vi "SelectAndResizeImageForFitting.vi"(0 "IMAQ Actual Image":T3, 1 "IMAQ Fitting Image":T3, 2 "ImageDisplay Refnum":refnum<vi>, 3 "Select Gaussian \nFit Methode":T1(ring), 4 "Subsampling":i32(ring)=16 items=["1"=1, "2"=2, "4"=4, "8"=8, "16"=16], 5 "error in":errorcluster, 6 "SimulationParameters":dbl[](array[slide])=[97.19626168224299, 38.62928348909657, 51.09034267912772, 14.330218068535824, 24.922118380062305, 127.10280373831775] caption="Amplitude\n\n\nX-Position\n\n\nY-Position\n\n\nWidth A\n\n\nWidth B\n\n\nAngle" scale=0.0..200.0, 7 "Cyclic Calculation Refnum":refnum<vi>, 9 "Image Busy Refnum":refnum<vi>) -> (13 "disable fit":bool, 14 "IMAQ Fitting Image Out":T3, 15 "FittingImageArray":dbl[][](array[numeric]), 16 "X samples":i32, 17 "Y samples":i32, 18 "ROI Offset":i32[](array[numeric]), 19 "error out":errorcluster)   [LabVIEW 2015]
uses:
  <vilib>/vision/Image Controls.llb/IMAQ Image.ctl
  <vilib>/vision/NI_Vision_Development_Module.lvlib
panel:
  out "ROI":T2
  in  "num X samples":i32=120
  in  "num Y samples":i32=100
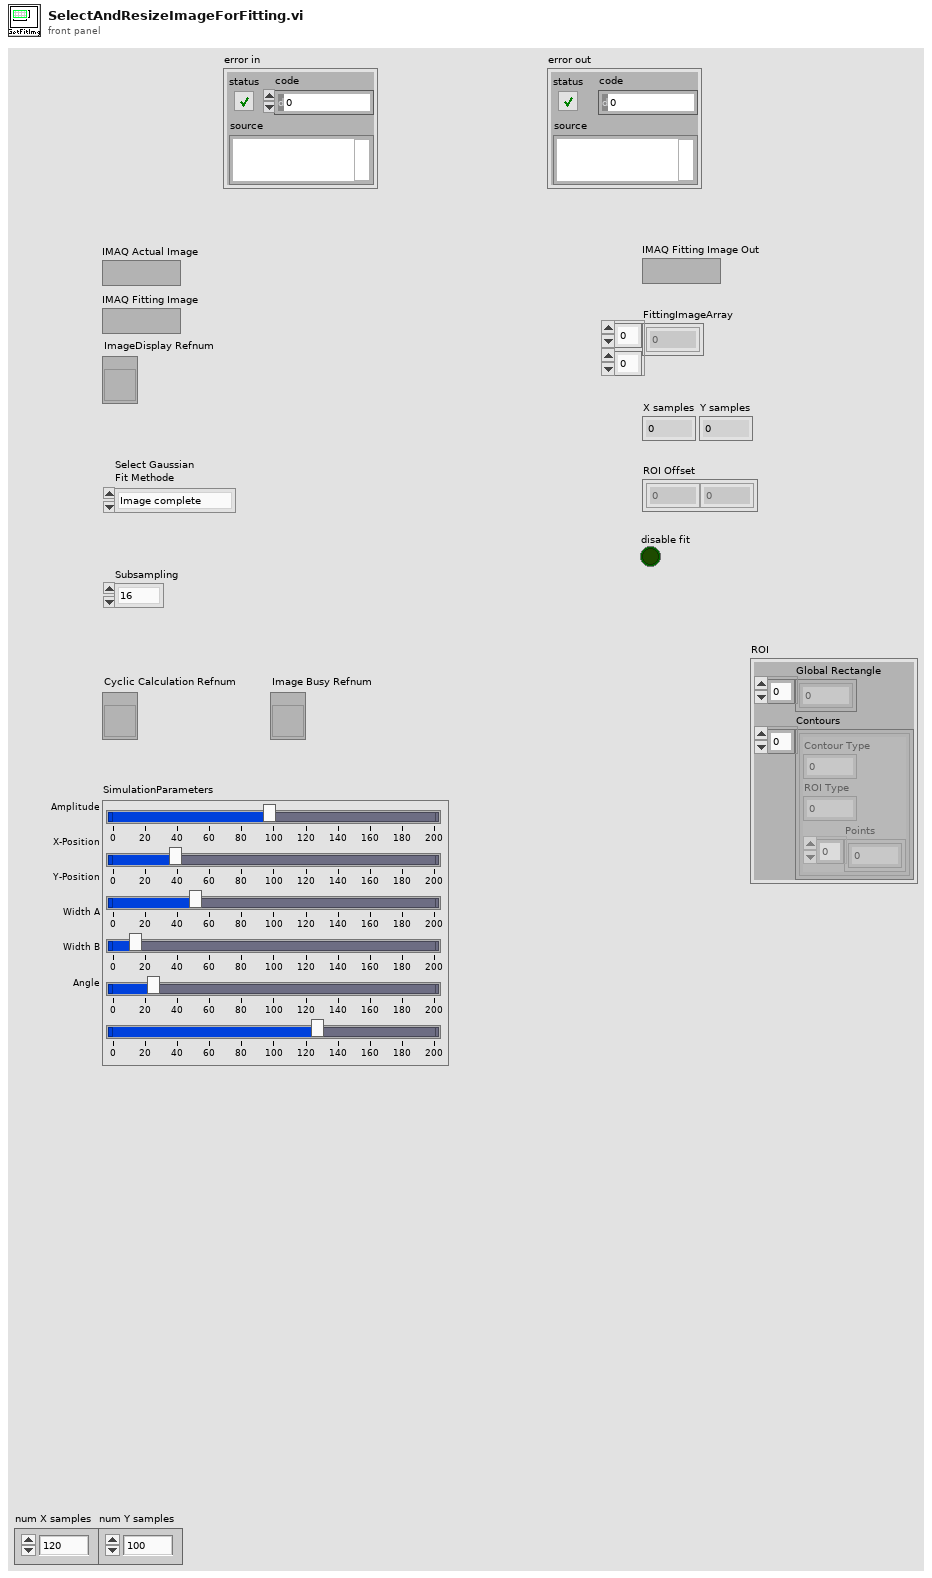
[diagram p1: front panel]
types:
  T1 = enum16{"Image complete", "Image with ROI", "AutoROI", "Simulation"}
  T2 = cluster{"Global Rectangle":i32[], "Contours":cluster{"Contour Type":u32, "ROI Type":u32, "Points":i32[]}[]}
  T3 = typedef "IMAQ Image.ctl" = refnum<image>
  T4 = typedef "IMAQ Rectangle" = cluster{"Left":i32, "Top":i32, "Right":i32, "Bottom":i32, "Rotation":dbl}
  T5 = cluster{"num X samples":i32, "num Y samples":i32}
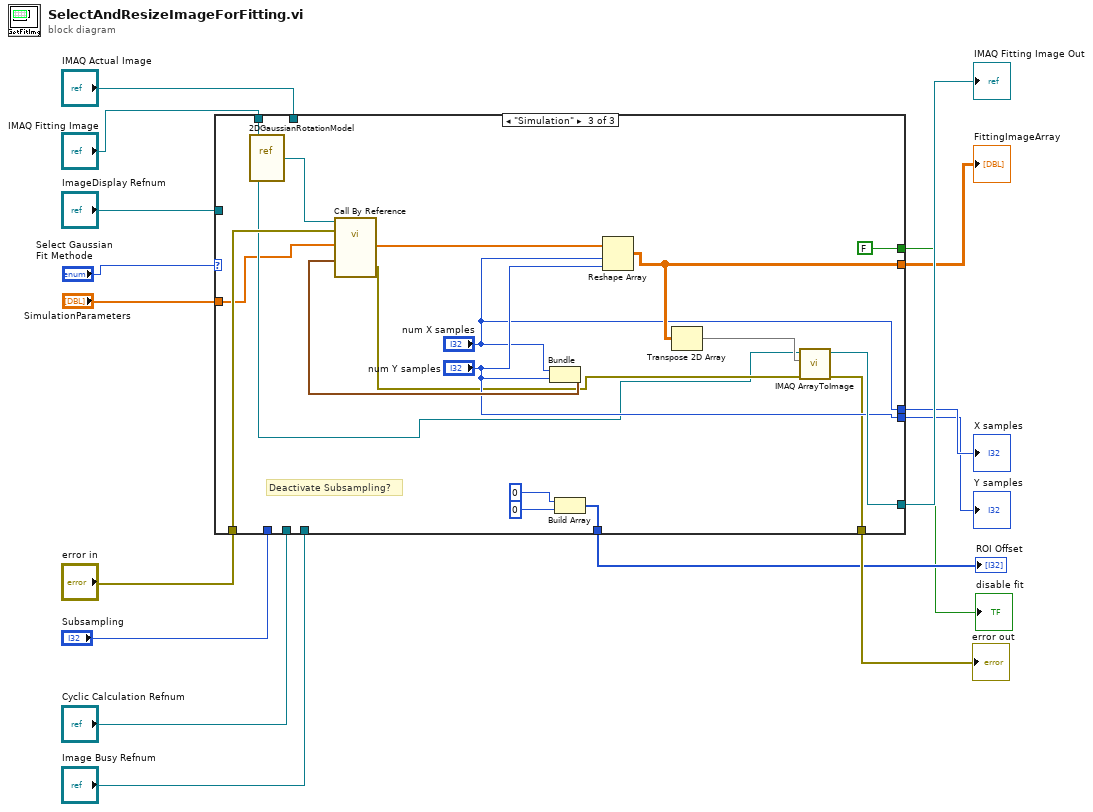
[diagram p0: block diagram]
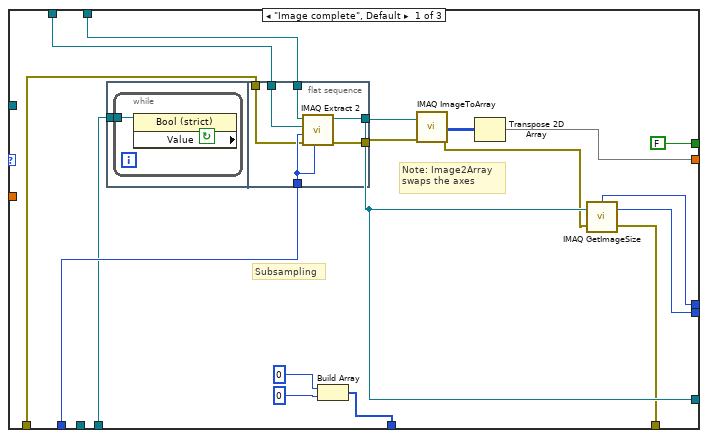
[diagram p2: hidden frame]
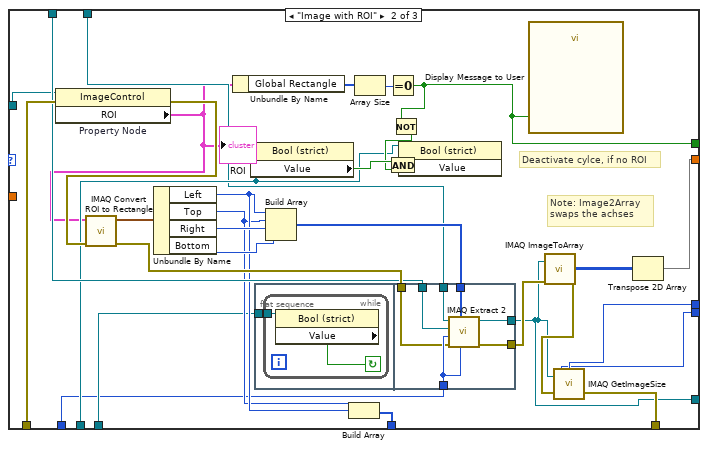
[diagram p3: hidden frame]
diagram:
  n1 = case shown="\"Simulation\"" "Select Gaussian \nFit Methode" {
    tunnel: [w32 w73 "num X samples"] -> w8
    tunnel: [w31 w72 "num Y samples"] -> w7
    tunnel: [w26 w71 w97] -> w6
    tunnel: [w30 w44 w95] -> w9
    tunnel: [w27 w70 w91] -> w15
    tunnel: "error in" -> [w23 w68 w92]
    tunnel: "Subsampling" -> [w24 w47 _]
    tunnel: [FALSE w57 FALSE] -> w5
    tunnel: "IMAQ Fitting Image" -> [w22 w53 w89]
    tunnel: "SimulationParameters" -> [_ _ w87]
    tunnel: "IMAQ Actual Image" -> [w21 w46 _]
    tunnel: [w18 w50 w84] -> w10
    tunnel: "Image Busy Refnum" -> [w17 w49 _]
    tunnel: "Cyclic Calculation Refnum" -> [_ w48 _]
    tunnel: "ImageDisplay Refnum" -> [_ w45 _]
    frame "Image complete", Default {
      # "Subsampling"
      # "Note: Image2Array \nswaps the axes"
      n2 = flat-sequence {
        tunnel: w17 -> [w34]
        tunnel: w21 -> [w42]
        tunnel: [w41] -> w30
        tunnel: [w40] -> w29
        tunnel: w24 -> [w39]
        tunnel: w22 -> [w38]
        tunnel: w23 -> [w37]
        frame #0 {
          n3 = while {
            tunnel: w34 -> [w35]
            stop <- w36 continue-if-true
            n4 = property on="Property Node" class="Bool (strict)"(reference=w35) -> ("Value"=w36:bool)  [unwired: 1 in, 2 out]
          }
        }
        frame #1 {
          n5 = call "IMAQ Extract 2"("Y Step Size"=w39, "error in (no error)"=w37, "X Step Size"=w39, "Image Dst"=w38, "Image Src"=w42) -> ("error out"=w40:errorcluster, "Image Dst Out"=w41:T3)  [unwired: 5 in]
        }
      }
      n6 = Build Array(0 ("Left"), 0 ("Top")) -> (w18:i32[])
      n7 = call "IMAQ ImageToArray"("error in (no error)"=w29, "Image"=w30) -> ("error out"=w28:errorcluster, "Image Pixels (U8)"=w33:u8[][])  [unwired: 2 in, 3 out]
      n8 = Transpose 2D Array(2D array=w33) -> (transposed array=w26:u8[][])
      n9 = call "IMAQ GetImageSize"("Image"=w30, "error in (no error)"=w28) -> ("Y Resolution"=w31:i32, "X Resolution"=w32:i32, "error out"=w27:errorcluster)  [unwired: 2 in]
    }
    frame "Image with ROI" {
      # "Deactivate cylce, if no ROI"
      # "Note: Image2Array \nswaps the achses"
      n10 = property on="Property Node" class="ImageControl"(reference=w45, error in=w68) -> (error out=w69:errorcluster, "ROI"=w43:T2)  [unwired: 1 out]
      "ROI" <- w43
      n11 = call "IMAQ Convert ROI to Rectangle"("error in (no error)"=w69, "ROI Descriptor"=w43) -> ("error out"=w54:errorcluster, "Rectangle"=w56:T4)  [unwired: 7 in]
      n12 = Unbundle By Name(w56) -> ("Left"=w52:i32, "Top"=w51:i32, "Right"=w65:i32, "Bottom"=w66:i32)
      n13 = Unbundle By Name(w43) -> ("Global Rectangle"=w63:i32[])
      n14 = property on="Property Node" class="Bool (strict)"(reference=w48) -> ("Value"=w60:bool)  [unwired: 1 in, 2 out]
      n15 = flat-sequence {
        tunnel: w49 -> [w74]
        tunnel: w46 -> [w83]
        tunnel: [w82] -> w44
        tunnel: [w81] -> w61
        tunnel: w47 -> [w80]
        tunnel: w55 -> [w79]
        tunnel: w54 -> [w78]
        tunnel: w53 -> [w77]
        frame #0 {
          n16 = while {
            tunnel: w74 -> [w75]
            stop <- w76 continue-if-true
            n17 = property on="Property Node" class="Bool (strict)"(reference=w75) -> ("Value"=w76:bool)  [unwired: 1 in, 2 out]
          }
        }
        frame #1 {
          n18 = call "IMAQ Extract 2"("Y Step Size"=w80, "Optional Rectangle"=w79, "error in (no error)"=w78, "X Step Size"=w80, "Image Dst"=w77, "Image Src"=w83) -> ("error out"=w81:errorcluster, "Image Dst Out"=w82:T3)  [unwired: 4 in]
        }
      }
      n19 = Build Array(w52, w51, w65, w66) -> (w55:i32[])
      n20 = Build Array(w52, w51) -> (w50:i32[])
      n21 = Array Size(array=w63) -> (size(s)=w62:i32)
      n22 = Equal To 0?(x=w62) -> (x = 0?=w57:bool)
      n23 = Not(x=w57) -> (.not. x?=w58:bool)
      n24 = And(x=w60, y=w58) -> (x .and. y?=w59:bool)
      n25 = property on="Property Node" class="Bool (strict)"(reference=w48, "Value"=w59) -> ()  [unwired: 1 in, 2 out]
      n26 = call "Display Message to User"("Enable"=w57) -> ()  [unwired: 9 in, 2 out]
      n27 = call "IMAQ ImageToArray"("error in (no error)"=w61, "Image"=w44) -> ("error out"=w64:errorcluster, "Image Pixels (U8)"=w67:u8[][])  [unwired: 2 in, 3 out]
      n28 = call "IMAQ GetImageSize"("Image"=w44, "error in (no error)"=w64) -> ("Y Resolution"=w72:i32, "X Resolution"=w73:i32, "error out"=w70:errorcluster)  [unwired: 2 in]
      n29 = Transpose 2D Array(2D array=w67) -> (transposed array=w71:u8[][])
    }
    frame "Simulation" {
      # "Deactivate Subsampling?"
      n30 = vi-ref "2DGaussianRotationModel.vi"() -> (w98:refnum<vi>)
      n31 = Bundle("num X samples"="num X samples", "num Y samples"="num Y samples") -> (w100:T5)  [unwired: 1 out]
      n32 = call-by-ref "?"(reference=w98, error in=w92, "data"=w100, "a"=w87) -> ("error out"=w93:errorcluster, "f(X,a)"=w99:dbl[])  [unwired: 2 in, 3 out]
      n33 = Build Array(0 ("Left"), 0 ("Top")) -> (w84:i32[])
      n34 = Reshape Array(w99, "num X samples", "num Y samples") -> (w97:dbl[][])
      n35 = Transpose 2D Array(2D array=w97) -> (transposed array=w96:dbl[][])
      n36 = call "IMAQ ArrayToImage"("error in (no error)"=w93, "Image Pixels (U8)"=w96, "Image"=w89) -> ("error out"=w91:errorcluster, "Image Out"=w95:T3)  [unwired: 7 in]
    }
  }
  "error out" <- w15
  "ROI Offset" <- w10
  "IMAQ Fitting Image Out" <- w9
  "X samples" <- w8
  "Y samples" <- w7
  "FittingImageArray" <- w6
  "disable fit" <- w5
